vi "Menu Item Clicked.vi"(8 "error in (no error)":errorcluster, 10 "menuItem":string, 11 "MainWindow in":refnum<class "MainWindow.lvclass">) -> (0 "error out":errorcluster, 3 "MainWindow out":refnum<class "MainWindow.lvclass">)   [LabVIEW 2020, in "MainWindow.lvlib" / "MainWindow.lvclass"]
uses:
  MainWindow.lvclass
  MainWindow.lvclass/MainWindow.ctl
  <vilib>/MGI/Panel Manager/Panel/Panel/Subpanel/Subpanel.lvclass
  C:/Program Files (x86)/National Instruments/LabVIEW 2020/vi.lib/MGI/Panel Manager/Panel/Panel/Panel.lvclass
  <vilib>/MGI/Panel Manager/Panel Actor/Panel Actor Messages/Change Panel Msg/Change Panel Msg.lvclass
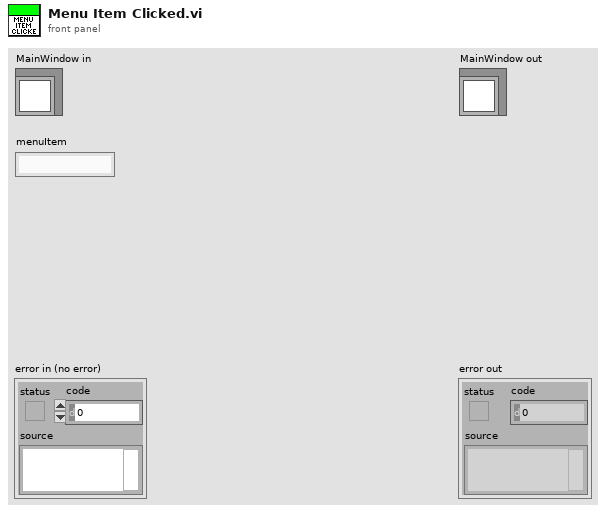
[diagram p1: front panel]
types:
  T1 = map{string, refnum<class "Message Enqueuer.lvclass">}
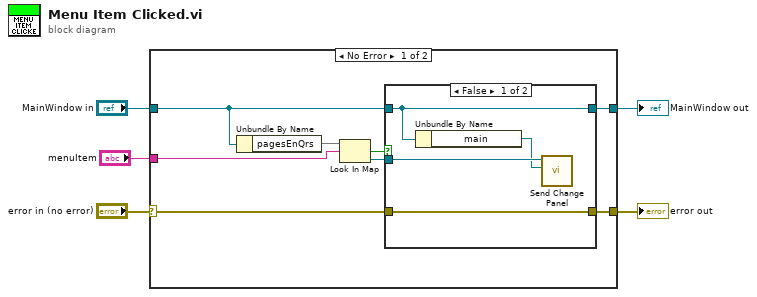
[diagram p0: block diagram]
diagram:
  n1 = case shown="No Error" "error in (no error)" {
    selector: "error in (no error)" -> [w9 w21]
    tunnel: [w10 w21] -> w4
    tunnel: [w8 w20] -> w2
    tunnel: "MainWindow in" -> [w7 w20]
    tunnel: "menuItem" -> [w12 _]
    frame No Error {
      n2 = Unbundle By Name(w7) -> ("pagesEnQrs"=w13:T1)
      n3 = Look In Map(map=w13, key=w12) -> (key not found?=w11:bool, value=w6:refnum<class "Message Enqueuer.lvclass">)  [unwired: 1 in]
      n4 = case shown="False" w11 {
        tunnel: [w17 w19] -> w10
        tunnel: w9 -> [w17 w19]
        tunnel: [w15 w18] -> w8
        tunnel: w7 -> [w15 w18]
        tunnel: w6 -> [w16 _]
        frame False {
          n5 = Unbundle By Name(w15) -> ("main"=w14:refnum<class "Subpanel.lvclass">)
          n6 = call <vilib>:"Send Change Panel.vi"("New Panel"=w14, "Message Enqueuer in"=w16) -> ()  [unwired: 8 in, 2 out]
        }
        frame True {
        }
      }
    }
    frame Error {
    }
  }
  "error out" <- w4
  "MainWindow out" <- w2
